vi "Save Data INT.vi"(4 "transpose? (no:F)":bool=TRUE, 6 "Initialize?":bool, 7 "Generate Index":bool=TRUE, 8 "error in (no error)":errorcluster, 9 "Data":i16[][](array[numeric]), 10 "Save data details":T1={"Data file path"=path "", "Comments file path"=path "", "Channel names"=["Frequency", "Signal_X", "Signal_Y", "IF_X", "IF_Y"]}, 11 "Save data settings":T2={"Save data"=TRUE, "Data Root Path"=path "D:/Data", "File Prefix"="", "File Format"=enum."ASCII", "Save column names"=TRUE, "File Comments"="<Description of the current file>", "User/Prj"="<User Name/Project Description>"}) -> (0 "error out":errorcluster, 2 "Save data details out":T1)   [LabVIEW 2015]
uses:
  Controls/Save data settings.ctl
  Controls/File formats.ctl
  Controls/Save data details.ctl
  Append Data INT.vi
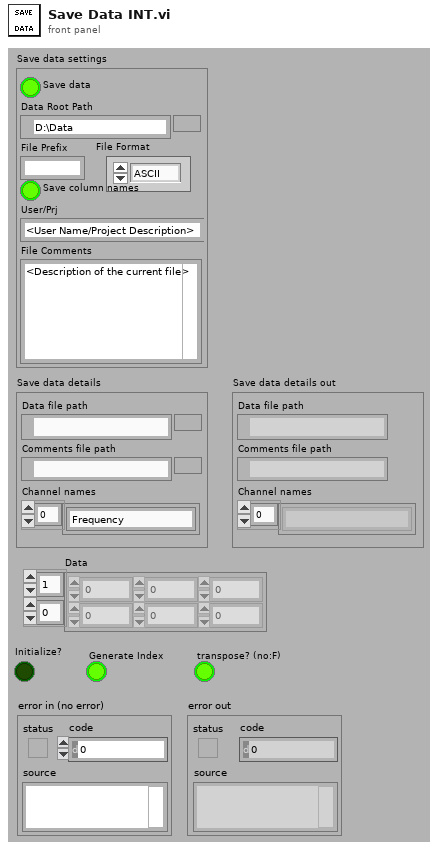
[diagram p1: front panel]
types:
  T1 = typedef "Save data details.ctl" = cluster{"Data file path":path, "Comments file path":path, "Channel names":string[]}
  T2 = typedef "Save data settings.ctl" = cluster{"Save data":bool, "Data Root Path":path, "File Prefix":string, "File Format":T3, "Save column names":bool, "File Comments":string, "User/Prj":string}
  T3 = typedef "File formats.ctl" = enum16{"TDMS", "ASCII", "BINARY"}
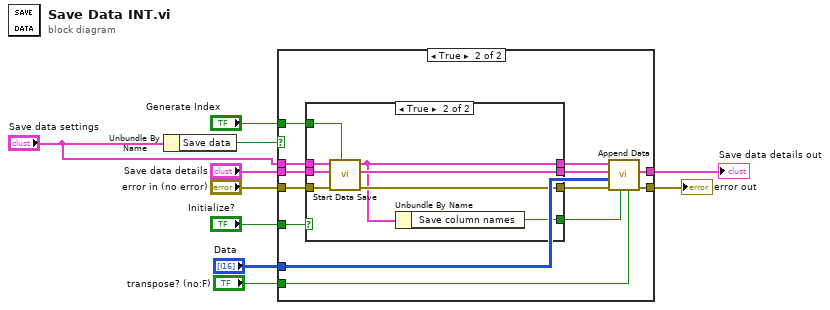
[diagram p0: block diagram]
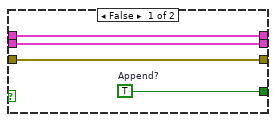
[diagram p3: hidden frame]
diagram:
  n1 = Unbundle By Name("Save data settings") -> ("Save data"=w8:bool)
  n2 = case shown="True" w8 {
    tunnel: [w12 w22] -> w10
    tunnel: "error in (no error)" -> [w12 w25]
    tunnel: "Data" -> [_ w20]
    tunnel: "Save data details" -> [w11 w24]
    tunnel: [w11 w19] -> w5
    tunnel: "Initialize?" -> [_ w17]
    tunnel: "Save data settings" -> [_ w16]
    tunnel: "Generate Index" -> [_ w14]
    tunnel: "transpose? (no:F)" -> [_ w13]
    frame False {
    }
    frame True {
      n3 = case shown="True" w17 {
        tunnel: w25 -> [w27 w35]
        tunnel: w24 -> [w28 w36]
        tunnel: [w27 w34] -> w23
        tunnel: [w28 w33] -> w21
        tunnel: [w26 w30] -> w18
        tunnel: w16 -> [w29 w37]
        tunnel: [w29 w31] -> w15
        tunnel: w14 -> [_ w32]
        frame False {
          w26 = TRUE  # Append?
        }
        frame True {
          n4 = call "Start Data Save.vi"("Generate Index"=w32, "error in (no error)"=w35, "Save data details"=w36, "Save data settings"=w37) -> ("error out"=w34:errorcluster, "Save data details out"=w33:T1, "Save data settings out"=w31:T2)  [unwired: 5 in]
          n5 = Unbundle By Name(w31) -> ("Save column names"=w30:bool)
        }
      }
      n6 = call-poly "Append Data.vi"("transpose? (no:F)"=w13, "append to file? (new file:F)"=w18, "error in (no error)"=w23, "Data"=w20, "Save data details"=w21, "Save data settings"=w15) -> ("error out"=w22:errorcluster, "Save data details out"=w19:T1)  [unwired: 4 in]
    }
  }
  "error out" <- w10
  "Save data details out" <- w5
